vi "test Get Busspeed Nominal.vi"(11 "Test Case In":refnum<class "Test PCANBasic.lvclass">) -> (0 "error out":errorcluster, 3 "Test Case Out":refnum<class "Test PCANBasic.lvclass">)   [LabVIEW 2020, in "Test PCANBasic.lvclass"]
uses:
  Test PCANBasic.lvclass
  C:/Program Files/National Instruments/LabVIEW 2025/vi.lib/Astemes/LUnit/Test Case.lvclass
  <vilib>/Astemes/LUnit/Test Case.lvclass/Test Case.ctl
  source/PCANBasic.lvlib
  <vilib>/Astemes/LUnit/Test Case.lvclass
  Global PCAN Channel.vi
  Global PCAN Baudrate.vi
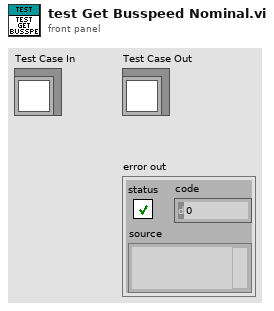
[diagram p1: front panel]
types:
  T1 = typedef "PCANBasic.lvlib/TPCANHandle.ctl" = u16
  T2 = typedef "PCANBasic.lvlib/PCAN Baud.ctl" = u16
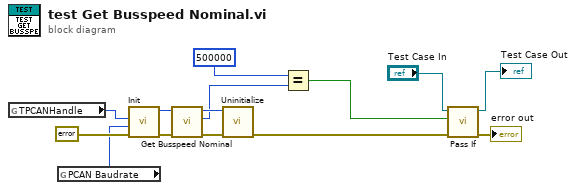
[diagram p0: block diagram]
diagram:
  n1 = global read "Global PCAN Channel.vi" "TPCANHandle"() -> (w8:T1)
  n2 = global read "Global PCAN Baudrate.vi" "PCAN Baudrate"() -> (w6:T2)
  n3 = call "Init.vi"("error in"=errorcluster {"status"=FALSE, "code"=0, "source"=""}, "Baudrate"=w6, "Channel"=w8) -> ("error out"=w9:errorcluster, "TPCANHandle out"=w7:T1)  [unwired: 6 in, 1 out]
  n4 = call "Get Busspeed Nominal.vi"("error in"=w9, "TPCANHandle in"=w7) -> ("error out"=w11:errorcluster, "Busspeed Nominal"=w3:u32, "TPCANHandle out"=w4:T1)  [unwired: 6 in, 1 out]
  n5 = call "Uninitialize.vi"("error in"=w11, "TPCANHandle in"=w4) -> ("error out"=w5:errorcluster)  [unwired: 8 in, 1 out]
  n6 = Equal?(x=u32 500000, y=w3) -> (x = y?=w1:bool)
  n7 = call <vilib>:"Pass If.vi"("error in (no error)"=w5, "Pass?"=w1, "LUnit Test Case In"="Test Case In") -> ("error out"=→"error out":errorcluster, "LUnit Test Case Out"=→"Test Case Out":refnum<class "Test PCANBasic.lvclass">)  [unwired: 7 in]
